vi "PXI-Enumerate AO Boards.vi"(8 "error in (no error)":errorcluster) -> (0 "error out":errorcluster, 1 "24-bit devices":tag[](array[tag]), 2 "Devices":tag[](array[tag]))   [LabVIEW 2020]
uses:
  <resource>/objmgr/daqmx.rc
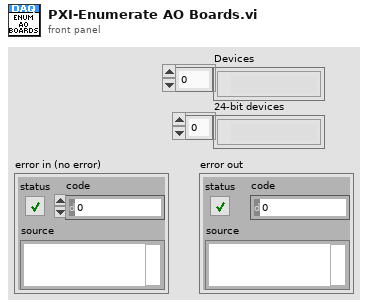
[diagram p1: front panel]
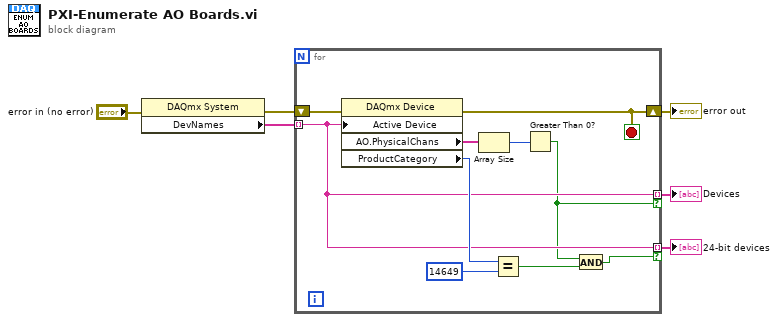
[diagram p0: block diagram]
diagram:
  n1 = property class="DAQmx System"(error in="error in (no error)") -> (error out=w6:errorcluster, "DevNames"=w5:tag[])  [unwired: 1 in, 1 out]
  n2 = for {
    tunnel: w5 -> [w10] mode=indexing
    shift-right: [w15] -> w3
    shift-left: w6 -> [w16]
    tunnel: [w10] -> w2 mode=indexing if=w8
    tunnel: [w10] -> w1 mode=indexing if=w7
    stop <- w15 stop-if-true
    n3 = property class="DAQmx Device"(error in=w16, "Active Device"=w10) -> (error out=w15:errorcluster, "AO.PhysicalChans"=w13:tag[], "ProductCategory"=w11:i32)  [unwired: 1 in, 1 out]
    n4 = Array Size(array=w13) -> (size(s)=w14:i32)
    n5 = Equal?(x=w11, y=14649) -> (x = y?=w9:bool)
    n6 = Greater Than 0?(x=w14) -> (x > 0?=w8:bool)
    n7 = And(x=w8, y=w9) -> (x .and. y?=w7:bool)
  }
  "error out" <- w3
  "Devices" <- w2
  "24-bit devices" <- w1
